vi "Launch Client Manager.vi"(8 "error in":errorcluster, 11 "System in":refnum<class "System.lvclass">) -> (0 "error out":errorcluster, 3 "System out":refnum<class "System.lvclass">)   [LabVIEW 2014, in "System.lvclass"]
uses:
  System.lvclass
  Client Child Classes/Client Manager/Client Manager.lvclass
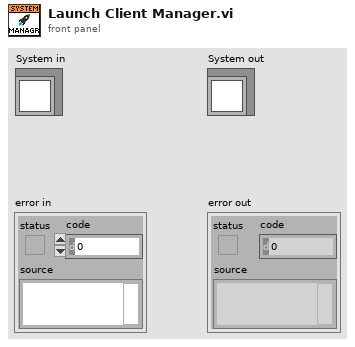
[diagram p1: front panel]
types:
  T1 = typedef "Client Ref.ctl" = cluster{"Name":string, "Path":path}
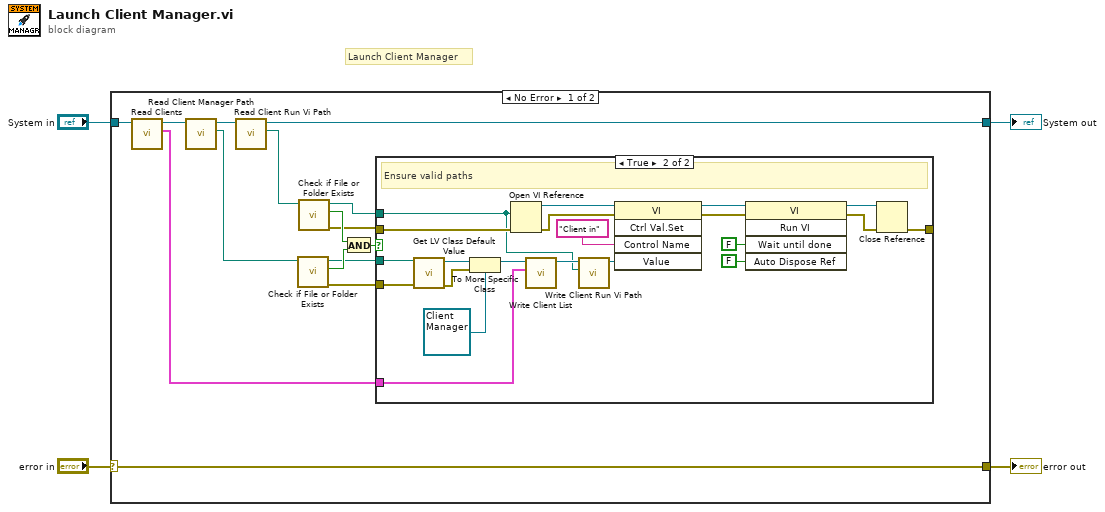
[diagram p0: block diagram]
diagram:
  # "Launch Client Manager"
  n1 = case shown="No Error" "error in" {
    selector: "error in" -> [w18 w43]
    tunnel: [w18 w43] -> w3
    tunnel: [w9 w42] -> w1
    tunnel: "System in" -> [w19 w42]
    frame No Error {
      n2 = call-dynamic "Read Clients.vi"("System in"=w19) -> ("Clients"=w5:T1[], "System out"=w6:refnum<class "System.lvclass">)  [unwired: 8 in, 1 out]
      n3 = call-dynamic "Read Client Manager Path.vi"("System in"=w6) -> ("Client Manager Path"=w7:path, "System out"=w10:refnum<class "System.lvclass">)  [unwired: 8 in, 1 out]
      n4 = call-dynamic "Read Client Run Vi Path.vi"("System in"=w10) -> ("Client Run Vi Path"=w8:path, "System out"=w9:refnum<class "System.lvclass">)  [unwired: 8 in, 1 out]
      n5 = call <vilib>:"Check if File or Folder Exists.vi"("path"=w7) -> ("error out"=w12:errorcluster, "file or folder exists?"=w16:bool, "dup path"=w11:path)  [unwired: 8 in]
      n6 = call <vilib>:"Check if File or Folder Exists.vi"("path"=w8) -> ("error out"=w14:errorcluster, "file or folder exists?"=w15:bool, "dup path"=w13:path)  [unwired: 8 in]
      n7 = And(x=w15, y=w16) -> (x .and. y?=w17:bool)
      n8 = case shown="True" w17 {
        tunnel: w11 -> [_ w37]
        tunnel: w12 -> [w20 w36]
        tunnel: [w20 w39] -> _
        tunnel: w13 -> [_ w21]
        tunnel: w14 -> [_ w33]
        tunnel: w5 -> [_ w23]
        frame False {
        }
        frame True {
          # "Ensure valid paths"
          n9 = call <vilib>:"Get LV Class Default Value.vi"("error in (no error)"=w36, "class path"=w37) -> ("error out"=w35:errorcluster, "object"=w38:refnum<class>)  [unwired: 8 in]
          n10 = To More Specific Class(target class=refnum<class "Client Manager.lvclass"> refnum ("Client Manager.lvclass"), reference=w38, error in=w35) -> (specific class reference=w34:refnum<class "Client Manager.lvclass">)  [unwired: 1 out]
          n11 = Open VI Reference(vi path=w21, error in (no error)=w33) -> (vi reference=w27:refnum<vi>, error out=w26:errorcluster)  [unwired: 4 in]
          n12 = call-dynamic "Write Client List.vi"("Client List"=w23, "Client Manager in"=w34) -> ("Client Manager out"=w25:refnum<class "Client Manager.lvclass">)  [unwired: 8 in, 1 out]
          n13 = call-dynamic "Write Client Run Vi Path.vi"("Client Run Vi Path"=w21, "Client Manager in"=w25) -> ("Client Manager out"=w22:refnum<class "Client Manager.lvclass">)  [unwired: 8 in, 1 out]
          n14 = invoke class="VI" method="Ctrl Val.Set"(reference=w27, error in=w26, "Control Name"="Client in" ("Client Name"), "Value"=w22) -> (reference out=w30:refnum<vi>, error out=w29:errorcluster)  [unwired: 1 in, 3 out]
          n15 = invoke class="VI" method="Run VI"(reference=w30, error in=w29, "Wait until done"=FALSE ("Wait Until Done"), "Auto Dispose Ref"=FALSE ("Auto Dispose Reference")) -> (reference out=w41:refnum<vi>, error out=w40:errorcluster)  [unwired: 1 in, 3 out]
          n16 = Close Reference(reference=w41, error in (no error)=w40) -> (error out=w39:errorcluster)
        }
      }
    }
    frame Error {
    }
  }
  "error out" <- w3
  "System out" <- w1
